vi "Hardware-DI-IPhaseLearn-Host.vi"() -> ()   [LabVIEW 2016]
panel:
  in  "TargetProfile":sgl[][](array[numeric])
  out "_TargetProfileSave":string[][](array[string])
  in  "DIChannel":T1(ring)
  in  "PiezoQLearn":bool
  out "ChgRSquare":sgl
  in  "FitThreshold":sgl=-1.0
  out "DischgRSquare":sgl
  in  "DischgShift":i32=-1
  in  "ChgShift":i32=-1
  in  "MaxAdj":sgl caption="[s]" format="%#_6p"
  in  "MinAdj":sgl caption="[s]" format="%#_6p"
  in  "Enable":bool caption="Learn Mode"
  in  "Kp":sgl caption="[s/unit]" format="%#_6p"
  in  "Init":bool
  out "ScopeV":sgl[](array[numeric])
  in  "Filepath":string
  out "HW|DI-Scope|dt":sgl
  in  "_Refresh":bool
  in  "_Save":bool
  in  "_Filepath":path caption="Target Profile Filepath (Local)"
  in  "_TargetProfile":string[][](table) caption="Target Profile"
  out "ScopeQ":sgl[](array[numeric])
  out "ScopeI":sgl[](array[numeric])
  out "DischgTarget":sgl[](array[numeric])
  out "DischgFdbk":sgl[](array[numeric])
  out "ChgFdbk":sgl[](array[numeric])
  out "ChgTarget":sgl[](array[numeric])
  out "_Summary":string[][](table) caption="Summary"
  out "_Plot":T2(graph)
  in  "OffsetI":sgl caption="[A]" format="%#_6p"
  in  "OffsetV":sgl caption="[V]" format="%#_6p"
  in  "FiltFreq":sgl caption="[Hz]" format="%#_6p"
  in  "Filter":enum16{"No Filter", "Butterworth"}(ring)
  in  "ScopeChannelI":i32(ring) caption="ScopeChannel" items=["Channel 1", "Channel 2", "Channel 3", "Channel 4"]
  in  "ScopeChannelV":i32(ring) caption="ScopeChannel" items=["Channel 1", "Channel 2", "Channel 3", "Channel 4"]
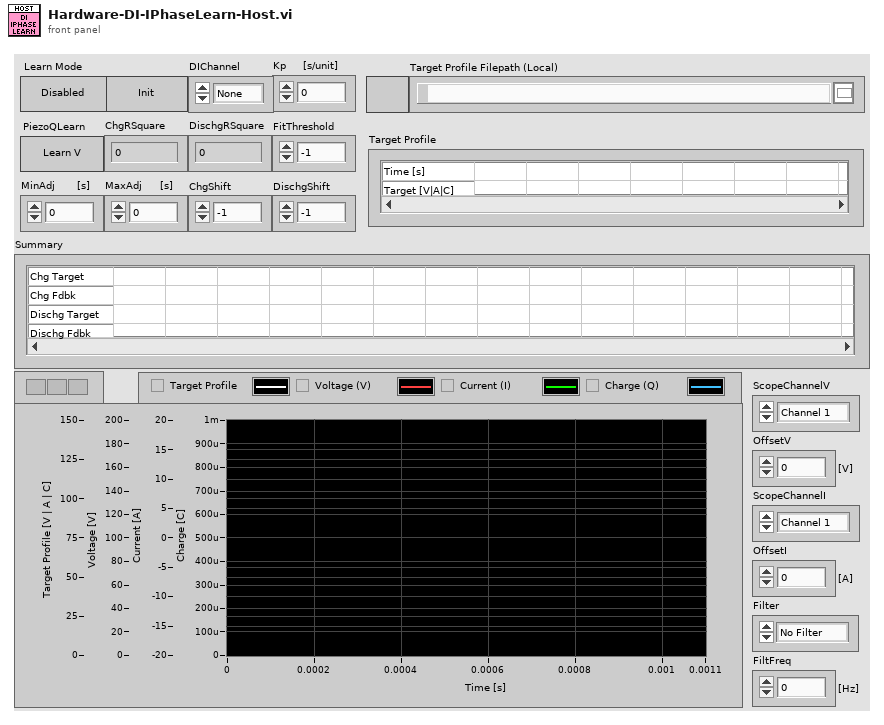
[diagram p1: front panel]
types:
  T1 = enum8{"None", "A1", "A2", "A3", "A4", "A5", "A6", "A7", "A8", "B1", "B2", "B3", "B4", "B5", "B6", "B7", "B8"}
  T2 = cluster{"TargetProfile":sgl[], "TargetProfile":sgl[]}[]
  T3 = cluster{"TargetProfile":sgl[], "TargetProfile":sgl[]}
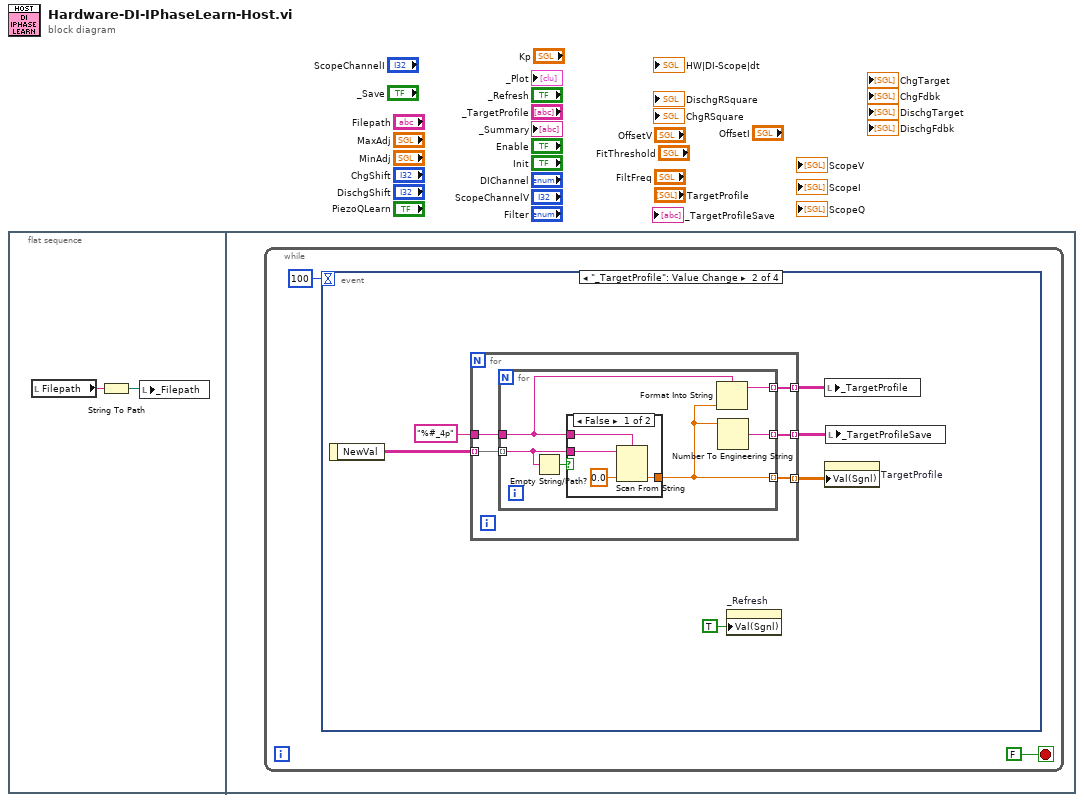
[diagram p0: block diagram]
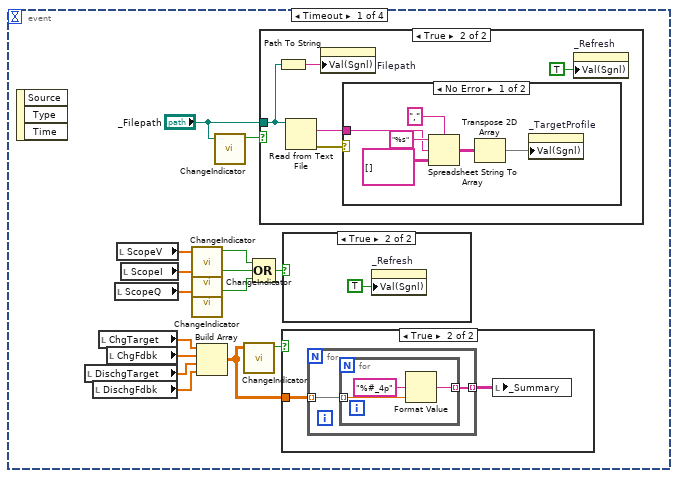
[diagram p2: hidden frame]
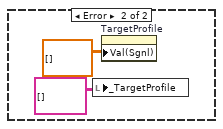
[diagram p4: hidden frame]
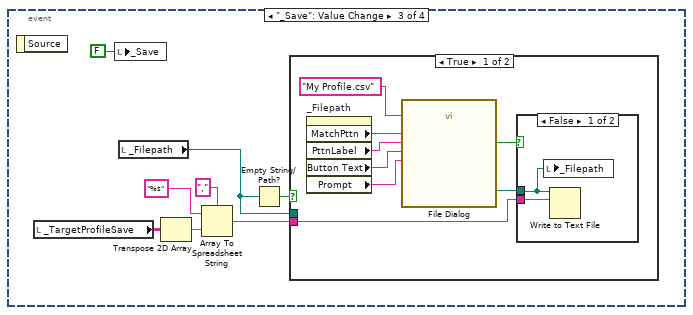
[diagram p8: hidden frame]
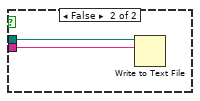
[diagram p10: hidden frame]
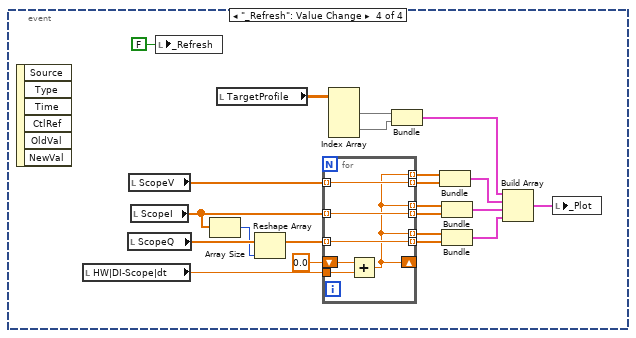
[diagram p11: hidden frame]
diagram:
  n1 = flat-sequence {
    frame #0 {
      n2 = local read "Filepath"() -> (w2:string)
      n3 = String To Path(string=w2) -> (path=w1:path)
      n4 = local write "_Filepath"(w1) -> ()
    }
    frame #1 {
      n5 = while {
        stop <- FALSE stop-if-true
        n6 = event shown="[1] \"_TargetProfile\": Value Change" {
          selector: _ -> [_ _ _ _]
          dyn-events: _ -> [_ _ _ _]
          timeout: 100 -> [_ _ _ _]
          event Timeout {
            n7 = event-data() -> ()  [unwired: 1 in, 3 out]
            n8 = local read "DischgTarget"() -> (w15:sgl[])
            n9 = local read "DischgFdbk"() -> (w14:sgl[])
            n10 = local read "ChgTarget"() -> (w19:sgl[])
            n11 = local read "ChgFdbk"() -> (w18:sgl[])
            n12 = local read "ScopeQ"() -> (w11:sgl[])
            n13 = local read "ScopeV"() -> (w13:sgl[])
            n14 = local read "ScopeI"() -> (w12:sgl[])
            n15 = call "ChangeIndicator.vi"("Input"=w13) -> ("Change"=w9:bool)  [unwired: 9 in]
            n16 = call "ChangeIndicator.vi"("Input"=w12) -> ("Change"=w10:bool)  [unwired: 9 in]
            n17 = call "ChangeIndicator.vi"("Input"=w11) -> ("Change"=w8:bool)  [unwired: 9 in]
            n18 = Build Array(w19, w18, w15, w14) -> (w17:sgl[][])
            n19 = call "ChangeIndicator.vi"("Input"="_Filepath") -> ("Change"=w5:bool)  [unwired: 9 in]
            n20 = call "ChangeIndicator.vi"("Input"=w17) -> ("Change"=w16:bool)  [unwired: 9 in]
            n21 = Compound Arithmetic op=OR(w9, w10, w8) -> (w7:bool)
            n22 = case shown="True" w5 {
              tunnel: "_Filepath" -> [_ w22]
              frame False {
              }
              frame True {
                n23 = Path To String(path=w22) -> (string=w24:string)
                n24 = Read from Text File(file (use dialog)=w22) -> (text=w21:string, error out=w20:errorcluster)  [unwired: 3 in, 2 out]
                n25 = property on="Filepath" class="Str"("Val(Sgnl)"=w24) -> ()  [unwired: 2 in, 2 out]
                n26 = case shown="No Error" w20 {
                  tunnel: w21 -> [w27 _]
                  frame No Error {
                    n27 = Spreadsheet String To Array(delimiter (Tab)=",", format string="%s", spreadsheet string=w27, array type (2D Dbl)=string[][] [] ("format string")) -> (array=w28:string[][])
                    n28 = Transpose 2D Array(2D array=w28) -> (transposed array=w26:string[][])
                    n29 = property on="_TargetProfile" class="Tbl (strict)"("Val(Sgnl)"=w26) -> ()  [unwired: 2 in, 2 out]
                  }
                  frame Error {
                    n30 = local write "_TargetProfile"(string[][] [] ("_TargetProfile")) -> ()
                    n31 = property on="TargetProfile" class="Arr (strict)"("Val(Sgnl)"=sgl[][] [] ("Value (Signaling)")) -> ()  [unwired: 2 in, 2 out]
                  }
                }
                n32 = property on="_Refresh" class="Bool (strict)"("Val(Sgnl)"=TRUE ("Value (Signaling)")) -> ()  [unwired: 2 in, 2 out]
              }
            }
            n33 = case shown="True" w16 {
              tunnel: w17 -> [_ w34]
              frame False {
              }
              frame True {
                n34 = for {
                  tunnel: w34 -> [w36] mode=indexing
                  tunnel: [w35] -> w33 mode=indexing
                  n35 = for {
                    tunnel: w36 -> [w39] mode=indexing
                    tunnel: [w37] -> w35 mode=indexing
                    n36 = Format Value(format string="%#_4p", value (0)=w39) -> (output string=w37:string)  [unwired: 1 in]
                  }
                }
                n37 = local write "_Summary"(w33) -> ()
              }
            }
            n38 = case shown="True" w7 {
              frame False {
              }
              frame True {
                n39 = property on="_Refresh" class="Bool (strict)"("Val(Sgnl)"=TRUE ("Value (Signaling)")) -> ()  [unwired: 2 in, 2 out]
              }
            }
          }
          event "_TargetProfile": Value Change {
            n40 = event-data() -> ("NewVal"=w44:string[][])  [unwired: 1 in]
            n41 = for {
              tunnel: "%#_4p" ("format string") -> [w51]
              tunnel: w44 -> [w50] mode=indexing
              tunnel: [w49] -> w43 mode=indexing
              tunnel: [w48] -> w42 mode=indexing
              tunnel: [w47] -> w41 mode=indexing
              n42 = for {
                tunnel: w51 -> [w52]
                tunnel: w50 -> [w57] mode=indexing
                tunnel: [w54] -> w49 mode=indexing
                tunnel: [w55] -> w48 mode=indexing
                tunnel: [w53] -> w47 mode=indexing
                n43 = Empty String/Path?(string/path=w57) -> (empty?=w56:bool)
                n44 = case shown="False" w56 {
                  tunnel: w52 -> [w61 _]
                  tunnel: [w60 _] -> w54
                  tunnel: w57 -> [w58 _]
                  frame False {
                    n45 = Scan From String(format string=w61, input string=w58, default 1=0.0 ("default value 1")) -> (output 1=w60:dbl)  [unwired: 2 in, 3 out]
                  }
                  frame True {
                  }
                }
                n46 = Format Into String(format string=w52, w54) -> (resulting string=w53:string)  [unwired: 2 in, 1 out]
                n47 = Number To Engineering String(4:w54) -> (0:w55:string)  [unwired: 3 in]
              }
            }
            n48 = property on="_Refresh" class="Bool (strict)"("Val(Sgnl)"=TRUE ("Value (Signaling)")) -> ()  [unwired: 2 in, 2 out]
            n49 = local write "_TargetProfile"(w41) -> ()
            n50 = property on="TargetProfile" class="Arr (strict)"("Val(Sgnl)"=w43) -> ()  [unwired: 2 in, 2 out]
            n51 = local write "_TargetProfileSave"(w42) -> ()
          }
          event "_Save": Value Change {
            n52 = event-data() -> ()  [unwired: 1 in, 1 out]
            n53 = local read "_TargetProfileSave"() -> (w68:string[][])
            n54 = local write "_Save"(FALSE ("_Save")) -> ()
            n55 = local read "_Filepath"() -> (w62:path)
            n56 = Transpose 2D Array(2D array=w68) -> (transposed array=w67:string[][])
            n57 = Array To Spreadsheet String(delimiter (Tab)=",", array=w67, 3:"%s" ("format string")) -> (spreadsheet string=w64:string)
            n58 = Empty String/Path?(string/path=w62) -> (empty?=w63:bool)
            n59 = case shown="True" w63 {
              tunnel: w64 -> [w77 w81]
              tunnel: w62 -> [_ w80]
              frame True {
                n60 = property on="_Filepath" class="Path"() -> ("MatchPttn"=w76:string, "PttnLabel"=w75:string, "Button Text"=w74:string, "Prompt"=w73:string)  [unwired: 2 in, 2 out]
                n61 = call "File Dialog"("prompt"=w73, "button label"=w74, "default name"="My Profile.csv", "pattern (all files)"=w76, "pattern label"=w75) -> ("selected path"=w72:path, "cancelled"=w70:bool)  [unwired: 7 in, 2 out]
                n62 = case shown="False" w70 {
                  tunnel: w77 -> [w79 _]
                  tunnel: w72 -> [w78 _]
                  frame False {
                    n63 = local write "_Filepath"(w78) -> ()
                    n64 = Write to Text File(file (use dialog)=w78, text=w79) -> ()  [unwired: 2 in, 3 out]
                  }
                  frame True {
                  }
                }
              }
              frame False {
                n65 = Write to Text File(file (use dialog)=w80, text=w81) -> ()  [unwired: 2 in, 3 out]
              }
            }
          }
          event "_Refresh": Value Change {
            n66 = event-data() -> ()  [unwired: 1 in, 6 out]
            n67 = local read "HW|DI-Scope|dt"() -> (w102:sgl)
            n68 = local read "ScopeQ"() -> (w89:sgl[])
            n69 = local read "ScopeV"() -> (w94:sgl[])
            n70 = local read "ScopeI"() -> (w82:sgl[])
            n71 = local write "_Refresh"(FALSE ("_Refresh")) -> ()
            n72 = Array Size(array=w82) -> (size(s)=w83:i32)
            n73 = local read "TargetProfile"() -> (w100:sgl[][])
            n74 = Reshape Array(w89, w83) -> (w84:sgl[])
            n75 = for {
              shift-right: [w104] -> _
              shift-left: sgl 0.0 -> [w109]
              tunnel: w102 -> [w108]
              tunnel: [w104] -> w96 mode=indexing
              tunnel: w94 -> [w107] mode=indexing
              tunnel: [w107] -> w95 mode=indexing
              tunnel: [w104] -> w92 mode=indexing
              tunnel: w82 -> [w106] mode=indexing
              tunnel: [w106] -> w93 mode=indexing
              tunnel: [w104] -> w91 mode=indexing
              tunnel: w84 -> [w105] mode=indexing
              tunnel: [w105] -> w90 mode=indexing
              # "dt is 25 ns"
              n76 = Add(x=w109, y=w108) -> (x+y=w104:sgl)
            }
            n77 = Index Array(array=w100) -> (element #1=w99:sgl[], element #2=w98:sgl[])  [unwired: 4 in]
            n78 = Bundle("TargetProfile"=w99, "TargetProfile"=w98) -> (w88:T3)  [unwired: 1 in]
            n79 = Bundle(w96, w95) -> (w87:cluster{sgl[], sgl[]})  [unwired: 1 in]
            n80 = Bundle(w92, w93) -> (w86:cluster{sgl[], sgl[]})  [unwired: 1 in]
            n81 = Bundle(w91, w90) -> (w85:cluster{sgl[], sgl[]})  [unwired: 1 in]
            n82 = Build Array(w88, w87, w86, w85) -> (w97:T2)
            n83 = local write "_Plot"(w97) -> ()
          }
        }
      }
    }
  }
